vi "Execute Set Boolean Type.vi"(6 "Mouse Position":T1, 8 "User VI Ref":refnum<vi>, 9 "Menu Item Tag Suffix":string, 10 "Remaining Items":refnum<vi>[](array[refnum]), 11 "Affected Items":T2) -> (0 "Fail transaction?":bool)   [LabVIEW 2021]
doc: "This VI will set a Boolean type that is input to the control's tag and stays persistent. It marks the data that is used in future application when changing themes.\n\n<b>Original</b>:This VI is part of a plug-in for modifying the LabVIEW shortcut menus. This is the execute VI which is called when the shortcut menu is chosen by the user. It performs the action of the selected menu item."
uses:
  Set Boolean Type.ctl
  <vilib>/Utility/miscctls.llb/LVPositionTypeDef.ctl
panel:
  # "All controls on this panel except \"Affected Items\" have been locked to prevent accidental edits. Changing the control names or types, other than the elements of the \"Affected Items\" cluster will make the VI unusable as a menu plugin.\n\nSee Context Help for each control for details about its use."
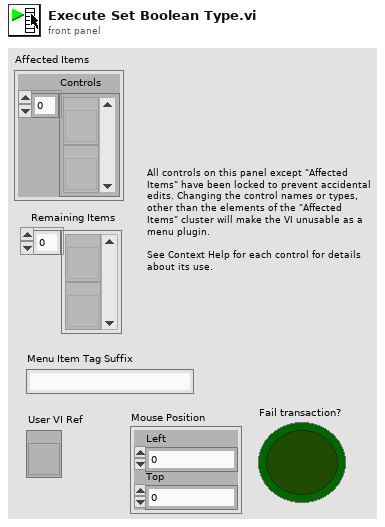
[diagram p1: front panel]
types:
  T1 = typedef "LVPositionTypeDef.ctl" = cluster{"Left":i32, "Top":i32}
  T2 = typedef "Set Boolean Type.ctl" = cluster{"Controls":refnum<vi>[]}
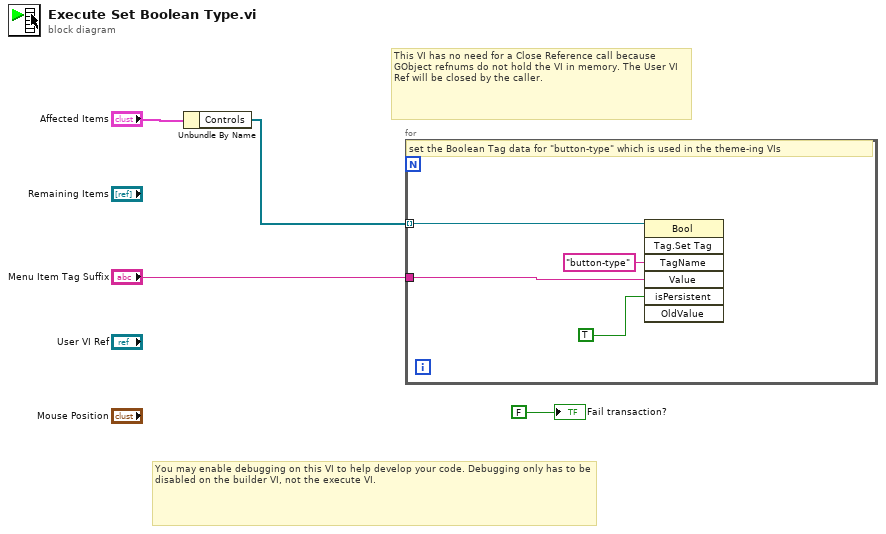
[diagram p0: block diagram]
diagram:
  # "You may enable debugging on this VI to help develop your code. Debugging only has to be disabled on the builder VI, not the execute VI."
  # "This VI has no need for a Close Reference call because GObject refnums do not hold the VI in memory. The User VI Ref will be closed by the caller."
  n1 = Unbundle By Name("Affected Items") -> ("Controls"=w2:refnum<vi>[])
  n2 = for {
    tunnel: w2 -> [w7] mode=indexing
    tunnel: "Menu Item Tag Suffix" -> [w5]
    # "set the Boolean Tag data for \"button-type\" which is used in the theme-ing VIs"
    n3 = invoke class="Bool" method="Tag.Set Tag"(reference=w7, "TagName"="button-type" ("Tag Name"), "Value"=w5, "isPersistent"=TRUE ("Is Persistent?")) -> ()  [unwired: 3 in, 7 out]
  }
  "Fail transaction?" <- FALSE ("Fail transaction?")
